vi "DRAM unpack data-test.vi"() -> ()   [LabVIEW 2015]
uses:
  <vilib>/rvi/Emulation/niFpgaGetClockAttributes.vi
  <vilib>/rvi/Emulation/niFpgaSctlEmulationGetInTimedLoop.vi
  <vilib>/rvi/Emulation/niFpgaEmulationReportErrorSimple.vi
  <vilib>/rvi/Emulation/niFpgaCriticalErrorInLSC.vi
panel:
  in  "packed data in":u32[](array[numeric])=[0, 0, 0, 0, 0, 0, 0, 0, 0, 0, 0, 0, 0, 0, 0, 0]
  in  "elements to read":i32
  out "output valid?":bool
  out "unpacked data out":u32
  in  "input valid":bool
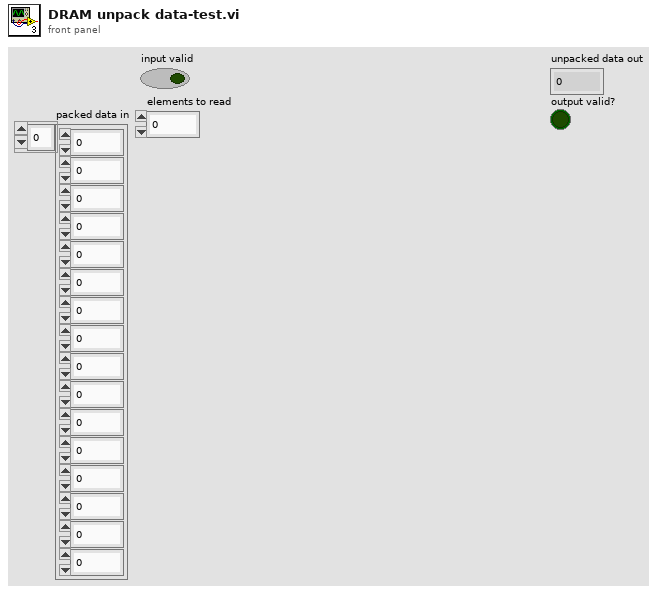
[diagram p1: front panel]
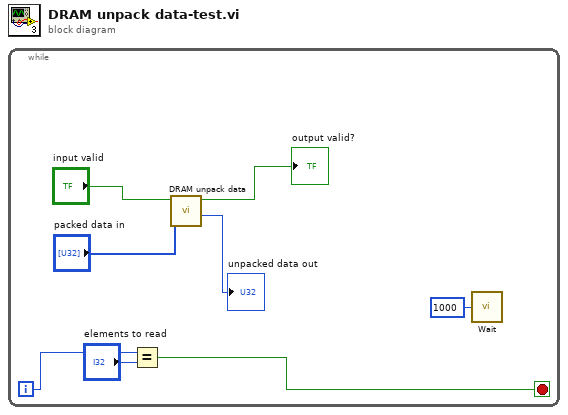
[diagram p0: block diagram]
diagram:
  n1 = while {
    i -> [w5]
    stop <- w3 stop-if-true
    n2 = Equal?(x=w5, y="elements to read") -> (x = y?=w3:bool)
    n3 = call "DRAM unpack data.vi"("packed data in"="packed data in", "input valid?"="input valid") -> ("unpacked data out"=→"unpacked data out":u32, "output valid?"=→"output valid?":bool)  [unwired: 8 in]
    n4 = call "Wait"("Count(mSec)"=u32 1000) -> ()  [unwired: 1 out]
  }
